vi "niRFSGPlayback Change Power and Freq.vi"(7 "Port":string, 8 "error in (no error)":errorcluster, 9 "LO configure setting":T1={"Carrier Frequency (Hz)"=5180000000.0, "Power Level(dBm)"=-10.0, "External Attenuation (dB)"=0.0} {"Carrier Frequency (Hz)" format="%#_6p"}, 11 "TSM Context":T2) -> (0 "error out":errorcluster {"code" format="%.0x"})   [LabVIEW 2014]
doc: "This example demonstrates generation of 802.11 single-channel waveform using an NI vector signal generator. The example reads the waveform from a TDMS file."
uses:
  <vilib>/NI_TestStand_SemiconductorModule/NI_TestStand_Semiconductor_Module.lvlibp/PinMap/General/SemiconductorModuleContext.ctl
  <vilib>/NI_TestStand_SemiconductorModule/NI_TestStand_Semiconductor_Module.lvlibp/PinMap/RF/RFPM/PinToNIRFPMSessions.vi
  <vilib>/NI_TestStand_SemiconductorModule/NI_TestStand_Semiconductor_Module.lvlibp/PinMap/RF/RFSG/PinToNIRFSGSession.vi
  <instrlib>/niRFPM/niRFPM.llb/NI-RFPM Fetch Source Offset By Parameters.vi
  <vilib>/NI_TestStand_SemiconductorModule/NI_TestStand_Semiconductor_Module.lvlibp
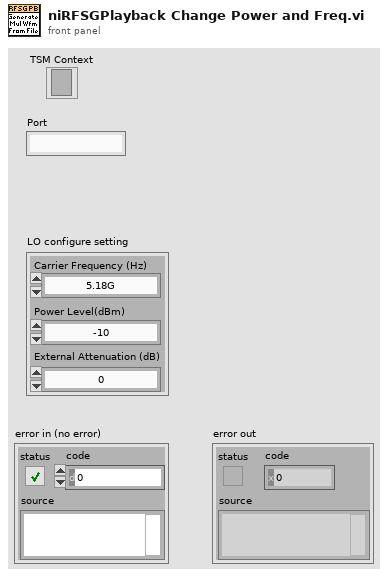
[diagram p1: front panel]
types:
  T1 = cluster{"Carrier Frequency (Hz)":dbl, "Power Level(dBm)":dbl, "External Attenuation (dB)":dbl}
  T2 = typedef "NI_TestStand_Semiconductor_Module.lvlibp/SemiconductorModuleContext.ctl" = refnum<k7>
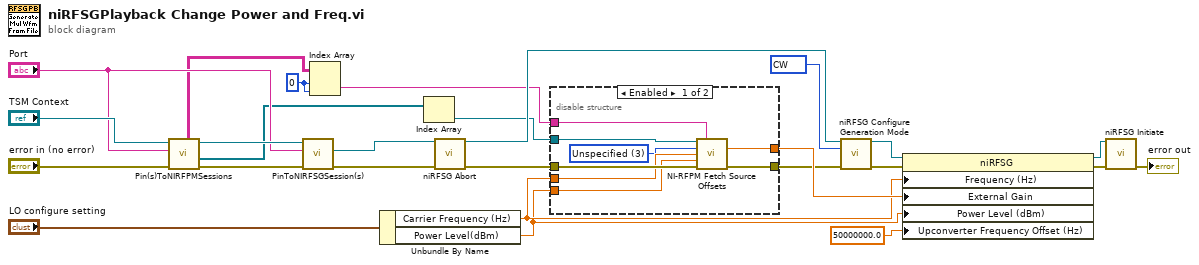
[diagram p0: block diagram]
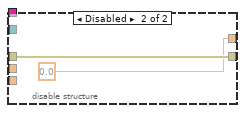
[diagram p2: hidden frame]
diagram:
  w4 = 0 ("index (row)")
  w18 = 1000 items=["CW"=1000, "Arb Waveform"=1001, "Script"=1002] ("generation mode")
  n1 = call-poly <vilib>:"Pin(s)ToNIRFPMSessions.vi"("error in (no error)"="error in (no error)", "Pin"="Port", "Semiconductor Module Context"="TSM Context") -> ("error out"=w3:errorcluster, "Instrument Sessions"=w2:refnum<k15>[], "Semiconductor Module Context out"=w9:T2, "Ports List"=w5:string[][])  [unwired: 3 in, 2 out]
  n2 = call-poly <vilib>:"PinToNIRFSGSession(s).vi"("error in (no error)"=w3, "Pin"="Port", "Semiconductor Module Context"=w9) -> ("error out"=w24:errorcluster, "Instrument Session"=w22:refnum<k15>)  [unwired: 5 in, 2 out]
  n3 = Index Array(array=w5, index (row)=w4, index (col)=w4) -> (element=w6:string)
  n4 = Unbundle By Name("LO configure setting") -> ("Carrier Frequency (Hz)"=w12:dbl, "Power Level(dBm)"=w11:dbl)
  n5 = Index Array(array=w2) -> (element=w1:refnum<k15>)  [unwired: 1 in]
  n6 = call <instrlib>:"niRFSG Abort.vi"("instrument handle"=w22, "error in"=w24) -> ("instrument handle out"=w17:refnum<k15>, "error out"=w23:errorcluster)  [unwired: 12 in]
  n7 = disable-structure shown="Enabled" {
    disable-tunnel: [w33 w36] -> w14
    disable-tunnel: [w32 0.0] -> w25
    disable-tunnel: w23 -> [w34 w36]
    disable-tunnel: w12 -> [w31 _]
    disable-tunnel: w11 -> [w30 _]
    disable-tunnel: w6 -> [w28 _]
    disable-tunnel: w1 -> [w27 _]
    frame Enabled {
      w29 = u32 3 items=["Unspecified"=3, "Loop"=2, "Gain"=1, "Direct"=0] ("Source Path")
      n8 = call-poly <instrlib>:"NI-RFPM Fetch Source Offsets.vi"("instrument handle"=w27, "Port"=w28, "Source Path"=w29, "frequency"=w31, "power"=w30, "error in"=w34) -> ("SourceOffset"=w32:dbl, "error out"=w33:errorcluster)  [unwired: 6 in, 2 out]
    }
    frame Disabled {
    }
  }
  n9 = call <instrlib>:"niRFSG Configure Generation Mode.vi"("instrument handle"=w17, "generation mode"=w18, "error in"=w14) -> ("instrument handle out"=w16:refnum<k15>, "error out"=w15:errorcluster)  [unwired: 11 in]
  n10 = property class="niRFSG"(reference=w16, error in=w15, "Frequency (Hz)"=w12, "External Gain"=w25, "Power Level (dBm)"=w11, "Upconverter Frequency Offset (Hz)"=50000000.0 ("Device Specific:Vector Signal Transceiver:Upconverter:Frequency Offset (Hz)")) -> (reference out=w20:refnum<k15>, error out=w19:errorcluster)
  n11 = call <instrlib>:"niRFSG Initiate.vi"("instrument handle"=w20, "error in"=w19) -> ("error out"=→"error out":errorcluster)  [unwired: 12 in, 1 out]
